vi "CreateSelfReference.vi"(8 "error in (no error)":errorcluster, 11 "Chart[Template]":refnum<class "Chart[Template].lvclass">) -> (0 "error out":errorcluster, 3 "Chart[Template] out":refnum<class "Chart[Template].lvclass">)   [LabVIEW 2019, in "Chart[Template].lvclass"]
doc: "JKI State Machine Objects (SMO) 1.0.0.5\nJKI - JKI\nCopyright (c) 2016, JKI"
uses:
  Chart[Template].lvclass
  Chart[Template].lvclass/Chart[Template].ctl
  vi.lib/JKI/JKI SMO/SMO.UI/SMO.UI.lvclass
  vi.lib/JKI/JKI SMO/SMO/SMO.lvclass
panel:
  # "For instructions on how to use the JKI State Machine Objects, examples and video tutorials, visit:\nhttp://jki.net/state-machine-objects/\n\nJKI State Machine Objects™\nhttp://jki.net/state-machine-objects/\nCopyright (C) 2005-2015, JKI <info@jki.net>\nALL RIGHTS RESERVED"
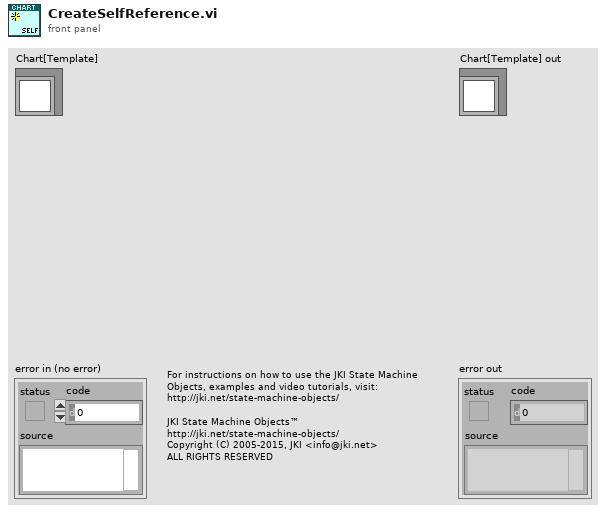
[diagram p1: front panel]
types:
  T1 = typedef "Chart[Template].lvclass/PrivateData--Ref.ctl" = refnum<data-value>
  T2 = typedef "Chart[Template].lvclass/PrivateData--Cluster.ctl" = cluster{"Public Events":T3, "Protected Events":T4, "Data":string, "Dependencies":T5}
  T3 = typedef "Chart[Template].lvclass/PublicEvents--Cluster.ctl" = cluster{"Chart cleared":refnum<user-event>}
  T4 = typedef "Chart[Template].lvclass/ProtectedEvents--Cluster.ctl" = cluster{"Clear Chart":refnum<user-event>}
  T5 = typedef "Chart[Template].lvclass/Dependencies--Cluster.ctl" = cluster{"SMO":refnum<class "SMO.lvclass">, "New Value":refnum<user-event>}
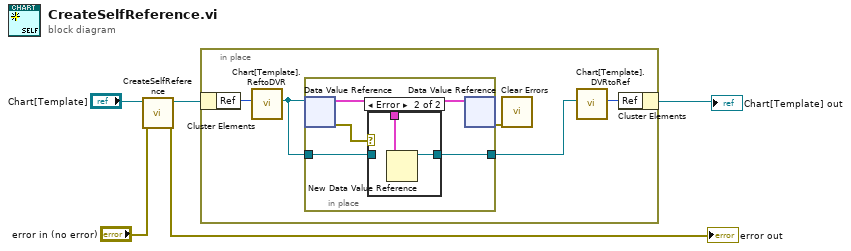
[diagram p0: block diagram]
diagram:
  n1 = call-parent "CreateSelfReference.vi"("error in (no error)"="error in (no error)", "SMO UI"="Chart[Template]") -> ("error out"=→"error out":errorcluster, "SMO UI out"=w4:refnum<class "Chart[Template].lvclass">)  [unwired: 8 in]
  n2 = in-place {
    n3 = in-place-cluster #1(w4) -> ("Ref"=w10:u32)
    n4 = call "Chart[Template].ReftoDVR.vi"("Ref"=w10) -> ("Ref"=w9:T1)  [unwired: 10 in]
    n5 = in-place {
      in-place-border: [w14] -> w7
      in-place-border: w9 -> [w11]
      n6 = in-place-dvr #2(w9) -> (w13:T2, w12:errorcluster)
      n7 = case shown="Error" w12 {
        tunnel: [w15 w17] -> w14
        tunnel: w13 -> [_ w16]
        tunnel: w11 -> [w15 _]
        frame No Error {
        }
        frame Error {
          n8 = New Data Value Reference(data value=w16) -> (data value reference=w17:refnum<data-value>)  [unwired: 1 in, 1 out]
        }
      }
      n9 = in-place-dvr #2(w13) -> (w6:errorcluster)  [unwired: 1 out]
    }
    n10 = call <vilib>:"Clear Errors.vi"("error in (no error)"=w6) -> ()  [unwired: 5 in, 2 out]
    n11 = call "Chart[Template].DVRtoRef.vi"("Ref"=w7) -> ("Ref"=w8:u32)  [unwired: 10 in]
    n12 = in-place-cluster #1("Ref"=w8) -> (→"Chart[Template] out":refnum<class "Chart[Template].lvclass">)
  }
